vi "setUpCRIOEnvironment.vi"() -> ()   [LabVIEW 2016]
uses:
  Typedefs/cRIO.ctl
  FileTransfer/FileTransfer.lvclass
  FileTransfer/FileTransfer.lvclass/FileTransfer.ctl
panel:
  out "error out":errorcluster
  in  "error in (no error)":errorcluster
  in  "cRIO":T1={"Username"="admin", "IP Address"="140.252.33.38", "Path to ts_opensplice target"=path "/usr", "Path to ts_sal target"=path "/usr"}
  in  "Linux Desktop":T2={"Username"="plotz", "IP Address"="127.0.0.1", "Path to ts_opensplice source"=path "/home/plotz/lsst_ts/ts_opensplice", "Path to ts_sal source"=path "/home/plotz/lsst_ts/ts_sal"}
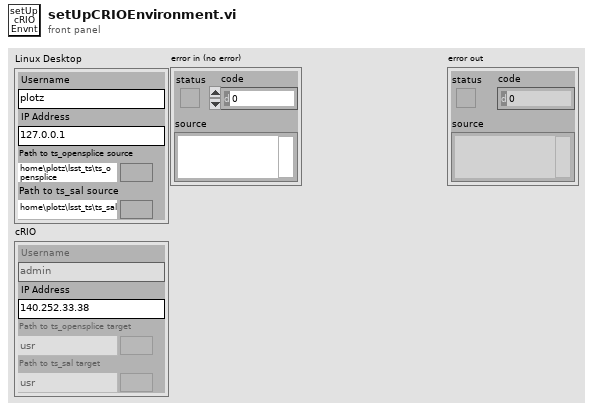
[diagram p1: front panel]
types:
  T1 = typedef "cRIO.ctl" = cluster{"Username":string, "IP Address":string, "Path to ts_opensplice target":path, "Path to ts_sal target":path}
  T2 = cluster{"Username":string, "IP Address":string, "Path to ts_opensplice source":path, "Path to ts_sal source":path}
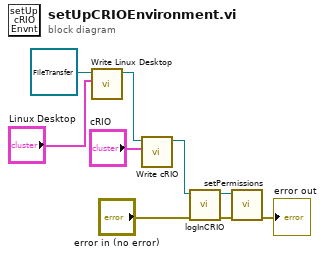
[diagram p0: block diagram]
diagram:
  n1 = call "Write Linux Desktop.vi"("Linux Desktop"="Linux Desktop", "FileTransfer in"=refnum<class "FileTransfer.lvclass"> refnum ("FileTransfer.lvclass")) -> ("FileTransfer out"=w8:refnum<class "FileTransfer.lvclass">)  [unwired: 9 in]
  n2 = call "Write cRIO.vi"("cRIO"="cRIO", "FileTransfer in"=w8) -> ("FileTransfer out"=w5:refnum<class "FileTransfer.lvclass">)  [unwired: 9 in]
  n3 = call "logInCRIO.vi"("error in (no error)"="error in (no error)", "FileTransfer in"=w5) -> ("error out"=w2:errorcluster, "FileTransfer out"=w3:refnum<class "FileTransfer.lvclass">)  [unwired: 8 in]
  n4 = call "setPermissions.vi"("error in (no error)"=w2, "FileTransfer in"=w3) -> ("error out"=→"error out":errorcluster)  [unwired: 8 in, 1 out]
